vi "16_6_Fxp_addation.vi"(1 "y":fxp<+/-,6,16>, 2 "x":fxp<+/-,6,16>) -> (0 "x+y":fxp<+/-,7,17> format="%.41g")   [LabVIEW 2020]
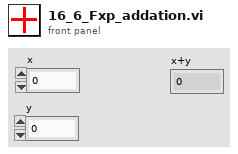
[diagram p1: front panel]
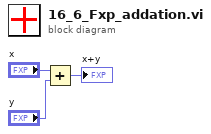
[diagram p0: block diagram]
diagram:
  n1 = Add(x="x", y="y") -> (x+y=→"x+y":fxp<+/-,7,17>)
